vi "Python_TransferFile.vi"(8 "File text":string, 9 "File name":string, 10 "Python version":string="3.9", 11 "Port":string) -> (2 "Console":string)   [LabVIEW 2022 SP3]
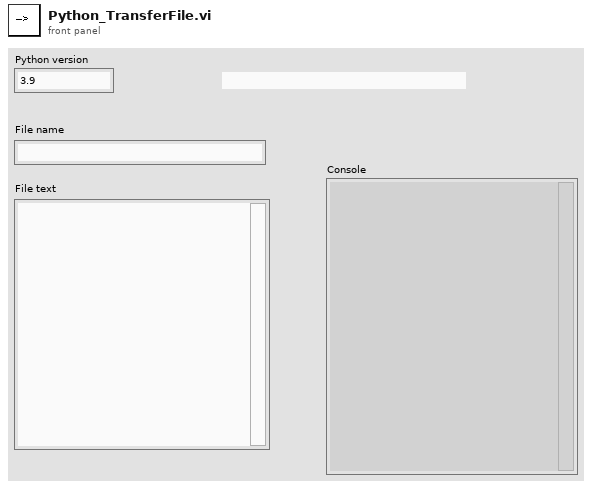
[diagram p1: front panel]
types:
  T1 = typedef "PythonCtrl.ctl" = cluster{"session":refnum<k35>, "PyPath":path, "Processor":T2, "Port":string, "version":string}
  T2 = typedef "Processors.ctl" = enum16{"SPIKE", "Pi", "Pi_ssh", "OpenMV", "Dunio"}
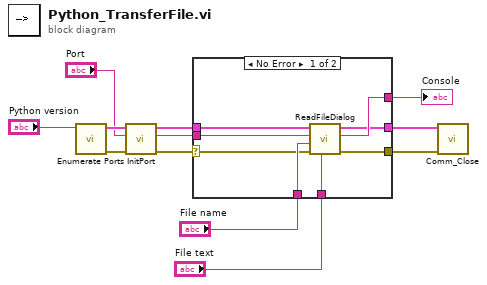
[diagram p0: block diagram]
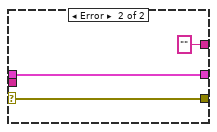
[diagram p2: hidden frame]
diagram:
  n1 = call "Enumerate Ports.vi"("Python version"="Python version") -> ("error out"=w10:errorcluster, "Python"=w12:T1)  [unwired: 5 in, 4 out]
  n2 = call "InitPort.vi"("error in (no error)"=w10, "Port"="Port", "Python"=w12) -> ("error out"=w3:errorcluster, "Console"=w7:string, "Python out"=w8:T1)  [unwired: 6 in]
  n3 = case shown="No Error" w3 {
    selector: w3 -> [w13 w20]
    tunnel: w8 -> [w16 w22]
    tunnel: w7 -> [w15 _]
    tunnel: "File name" -> [w19 _]
    tunnel: [w18 w20] -> w1
    tunnel: [w16 w22] -> w5
    tunnel: [w17 "" ("Console")] -> w4
    tunnel: "File text" -> [w14 _]
    frame No Error {
      n4 = call "ReadFileDialog.vi"("File Text"=w14, "error in (no error)"=w13, "File name"=w19, "Console in"=w15, "Python in"=w16) -> ("error out"=w18:errorcluster, "Console"=w17:string)  [unwired: 5 in]
    }
    frame Error {
    }
  }
  "Console" <- w4
  n5 = call "Comm_Close.vi"("error in (no error)"=w1, "Python in"=w5) -> ()  [unwired: 8 in, 2 out]
